vi "Configure Zero.vi"(8 "error in (no error)":errorcluster, 11 "VISA resource name":refnum<visa-resource-name>) -> (0 "error out":errorcluster, 3 "VISA resource name out":refnum<visa-resource-name>)   [LabVIEW 2017, in "RadWag balances and scales.lvlib"]
doc: "Zeros the balance (the tare value as well as displayed result is set to zero)."
uses:
  <instrlib>/Radwag Balances and Scales/Public/RadWag balances and scales.lvlib
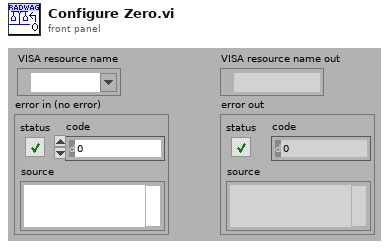
[diagram p1: front panel]
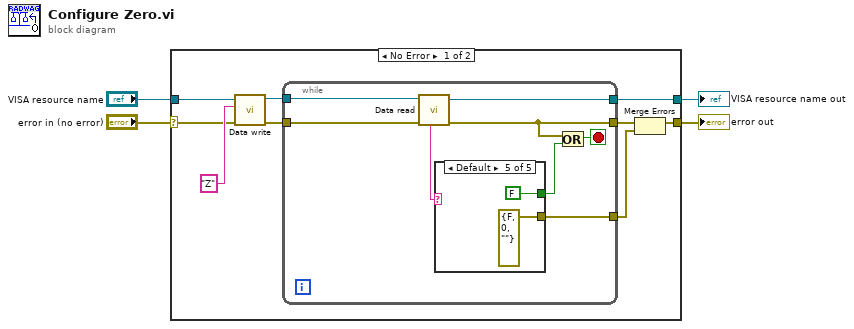
[diagram p0: block diagram]
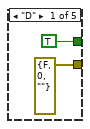
[diagram p2: hidden frame]
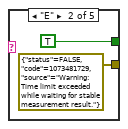
[diagram p3: hidden frame]
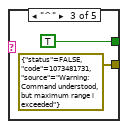
[diagram p4: hidden frame]
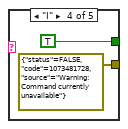
[diagram p5: hidden frame]
diagram:
  n1 = case shown="No Error" "error in (no error)" {
    selector: "error in (no error)" -> [w8 w32]
    tunnel: "VISA resource name" -> [w13 w33]
    tunnel: [w9 w33] -> w3
    tunnel: [w6 w32] -> w2
    frame No Error {
      n2 = call <instrlib>:"Data write.vi"("error in (no error)"=w8, "ID"="Z", "VISA resource name"=w13) -> ("error out"=w10:errorcluster, "VISA resource name out"=w11:refnum<visa-resource-name>)  [unwired: 7 in]
      n3 = while {
        tunnel: w11 -> [w21]
        tunnel: w10 -> [w20]
        tunnel: [w19] -> w9
        tunnel: [w17] -> w7
        tunnel: [w14] -> w5
        stop <- w18 stop-if-true
        n4 = call <instrlib>:"Data read.vi"("error in (no error)"=w20, "VISA resource name"=w21) -> ("error out"=w17:errorcluster, "VISA resource name out"=w19:refnum<visa-resource-name>, "Status"=w15:string)  [unwired: 3 in, 4 out]
        n5 = case shown="Default" w15 {
          tunnel: [TRUE TRUE TRUE TRUE FALSE] -> w16
          tunnel: [errorcluster {"status"=FALSE, "code"=0, "source"=""} ("error constant") errorcluster {"status"=FALSE, "code"=1073481729, "source"="Warning: Time limit exceeded while waiting for stable measurement result."} ("t") errorcluster {"status"=FALSE, "code"=1073481731, "source"="Warning: Command understood, but maximum range i exceeded"} ("t") errorcluster {"status"=FALSE, "code"=1073481728, "source"="Warning: Command currently unavailable"} ("t") errorcluster {"status"=FALSE, "code"=0, "source"=""} ("error constant")] -> w14
          frame "D" {
          }
          frame "E" {
          }
          frame "^" {
          }
          frame "I" {
          }
          frame Default {
          }
        }
        n6 = Or(x=w17, y=w16) -> (x .or. y?=w18:bool)
      }
      n7 = Merge Errors(w7, w5) -> (w6:errorcluster)
    }
    frame Error {
    }
  }
  "VISA resource name out" <- w3
  "error out" <- w2
